vi "New Observing Model.vi"() -> (1 "Test Reply Queue":refnum<queue>, 3 "ObservingModel Out":refnum<class "ObservingModel.lvclass">)   [LabVIEW 2017, in "TestPubSubRouting.lvlib" / "ObservingModel.lvclass"]
uses:
  ObservingModel.lvclass
  ObservingModel.lvclass/ObservingModel.ctl
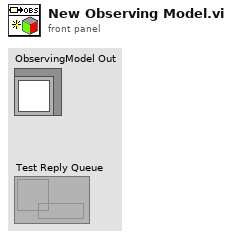
[diagram p1: front panel]
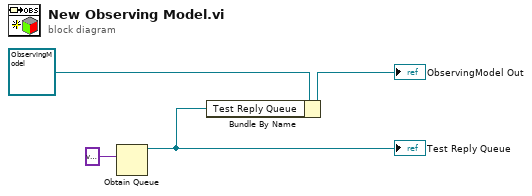
[diagram p0: block diagram]
diagram:
  n1 = Obtain Queue(element data type=variant) -> (queue out=w1:refnum<queue>)  [unwired: 4 in, 2 out]
  "Test Reply Queue" <- w1
  n2 = Bundle By Name(cluster=refnum<class "ObservingModel.lvclass"> refnum ("ObservingViewable in"), "Test Reply Queue"=w1) -> (→"ObservingModel Out":refnum<class "ObservingModel.lvclass">)
